vi "SRV_Sensor Streaming Sensors Off.vi"(0 "Previous Streaming Cfg-Cmds":T1[](array[typedef]) {"Calculated Sensors Array"."Parsed Formula"."Y Values" format="%.2f"; "Calculated Sensors Array"."Sensor Config"."Register" format="%.0x"; "Calculated Sensors Array"."Sensor Config"."I2C Address" format="%.0x"; "Calculated Sensors Array"."Sensor Config"."Sample Period (ms)" min=10 max=60000 step=1; "Calculated Sensors Array"."Sensor Config"."Digital Mask" format="%.0x"; "Calculated Sensors Array"."Sensor Config"."Channel" format="%.0x"; "Parsed Formula"."Y Values" format="%.2f"; "Sensor Config"."Register" format="%.0x"; "Sensor Config"."I2C Address" format="%.0x"; "Sensor Config"."Sample Period (ms)" min=10 max=60000 step=1; "Sensor Config"."Digital Mask" format="%.0x"; "Sensor Config"."Channel" format="%.0x"}, 11 "error in (no error)":errorcluster) -> (6 "Streaming Cfg-Cmds OFF":T1[](array[typedef]) {"Calculated Sensors Array"."Parsed Formula"."Y Values" format="%.2f"; "Calculated Sensors Array"."Sensor Config"."Register" format="%.0x"; "Calculated Sensors Array"."Sensor Config"."I2C Address" format="%.0x"; "Calculated Sensors Array"."Sensor Config"."Sample Period (ms)" min=10 max=60000 step=1; "Calculated Sensors Array"."Sensor Config"."Digital Mask" format="%.0x"; "Calculated Sensors Array"."Sensor Config"."Channel" format="%.0x"; "Parsed Formula"."Y Values" format="%.2f"; "Sensor Config"."Register" format="%.0x"; "Sensor Config"."I2C Address" format="%.0x"; "Sensor Config"."Sample Period (ms)" min=10 max=60000 step=1; "Sensor Config"."Digital Mask" format="%.0x"; "Sensor Config"."Channel" format="%.0x"}, 15 "error out":errorcluster)   [LabVIEW 2009]
uses:
  SRV_Sensor Config-Command Cluster.ctl
  SRV_Sensor Config Cluster.ctl
  SRV_Sensor Analog-Digital.ctl
  SRV_Sensor Sampling Mode.ctl
  SRV_Sensor View Config Cluster.ctl
  SRV_Sensors Names.ctl
  SRV_Sensor PicoC Shared Var Type.ctl
  SRV_Sensor Number of Bytes.ctl
  SRV_Sensor Integer Word Type.ctl
  SRV_Calculated Sensor Cfg.ctl
panel:
  # "operator"
  # "register1"
  # "register2"
  # "operator"
  # "register1"
  # "register2"
  # "operator"
  # "register1"
  # "register2"
  # "operator"
  # "register1"
  # "register2"
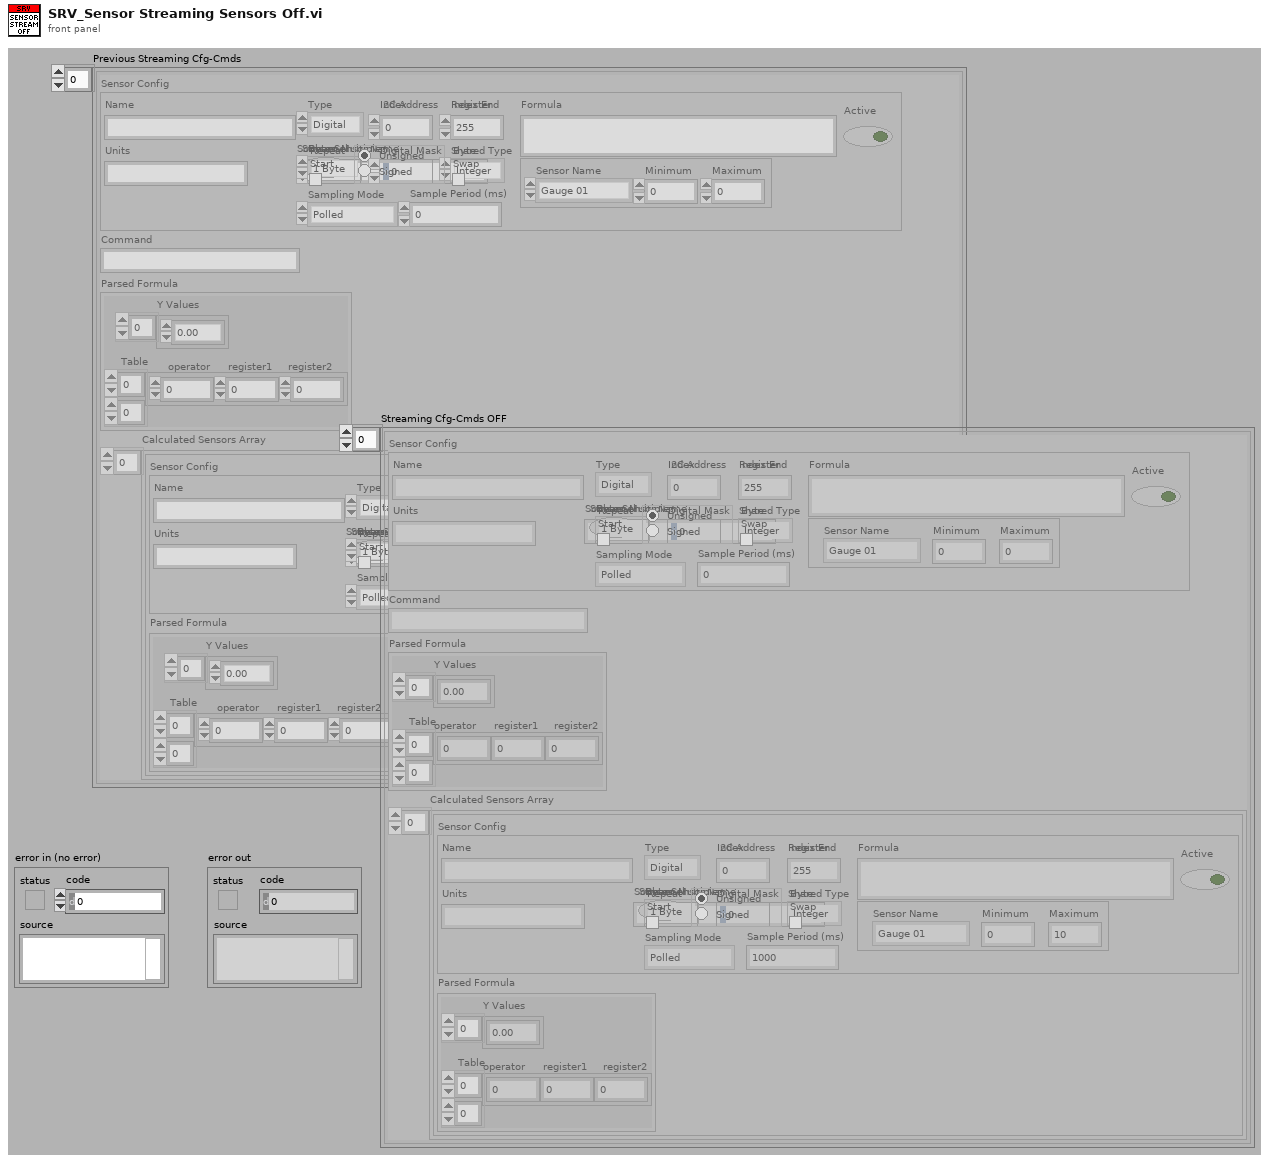
[diagram p1: front panel]
types:
  T1 = typedef "SRV_Sensor Config-Command Cluster.ctl" = cluster{"Sensor Config":T2, "Command":string, "Parsed Formula":cluster{"Table":i32[][], "Y Values":dbl[]}, "Calculated Sensors Array":T10[]}
  T2 = typedef "SRV_Sensor Config Cluster.ctl" = cluster{"Name":string, "A/D":T3, "I2C Address":u8, "Register":u8, "Channel":u8, "Digital Mask":u16, "Units":string, "Sampling Mode":T4, "Sample Period (ms)":u32, "Formula":string, "Sensor View Config":T5, "Active":bool, "PicoC Shared Var Type":T7, "Index":u8, "Stream Multiple?":bool, "Index End":u8, "Bytes":T8, "Source Sensor Name":string, "Repeat Start":bool, "Integer Word Type":T9, "Byte Swap":bool}
  T3 = typedef "SRV_Sensor Analog-Digital.ctl" = enum16{"Digital", "Analog", "PicoC Shared", "Calculated"}
  T4 = typedef "SRV_Sensor Sampling Mode.ctl" = enum16{"Polled", "Streaming"}
  T5 = typedef "SRV_Sensor View Config Cluster.ctl" = cluster{"Sensor Name":T6, "Minimum":dbl, "Maximum":dbl}
  T6 = typedef "SRV_Sensors Names.ctl" = enum16{"Gauge 01", "Gauge 02", "Gauge 03", "Gauge 04", "Meter 01", "Meter 02", "Meter 03", "Meter 04", "Numeric 01", "Numeric 02", "Numeric 03", "Numeric 04", "Numeric 05", "Numeric 06", "Numeric 07", "Numeric 08", "Boolean 01", "Boolean 02", "Boolean 03", "Boolean 04", "Boolean 05", "Boolean 06", "Boolean 07", "Boolean 08", "Boolean 09", "Boolean 10", "Boolean 11", "Boolean 12", "Boolean 13", "Boolean 14", "Boolean 15", "Boolean 16", "Boolean 17", "Boolean 18", "Boolean 19", "Boolean 20", "Boolean 21", "Boolean 22", "Boolean 23", "Boolean 24", "Boolean 25", "Boolean 26", "Boolean 27", "Boolean 28", "Boolean 29", "Boolean 30", "Boolean 31", "Boolean 32"}
  T7 = typedef "SRV_Sensor PicoC Shared Var Type.ctl" = enum16{"String", "Integer", "Float"}
  T8 = typedef "SRV_Sensor Number of Bytes.ctl" = enum16{"1 Byte", "2 Bytes"}
  T9 = typedef "SRV_Sensor Integer Word Type.ctl" = enum32{"Unsigned", "Signed"}
  T10 = typedef "SRV_Calculated Sensor Cfg.ctl" = cluster{"Sensor Config":T2, "Parsed Formula":cluster{"Table":i32[][], "Y Values":dbl[]}}
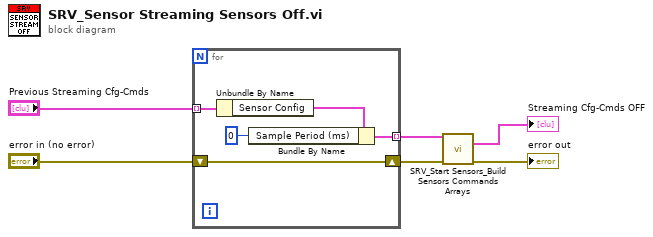
[diagram p0: block diagram]
diagram:
  n1 = for {
    tunnel: "Previous Streaming Cfg-Cmds" -> [w10] mode=indexing
    shift-right: [w8] -> w3
    shift-left: "error in (no error)" -> [w8]
    tunnel: [w7] -> w4 mode=indexing
    n2 = Unbundle By Name(w10) -> ("Sensor Config"=w9:T2)
    n3 = Bundle By Name(cluster=w9, "Sample Period (ms)"=u32 0 ("Sensor Config.Sample Period (ms)")) -> (w7:T2)
  }
  n4 = call "SRV_Start Sensors_Build Sensors Commands Arrays.vi"("Sensors Config"=w4, "error in (no error)"=w3) -> ("Active Streaming Cfg-Commands"=→"Streaming Cfg-Cmds OFF":T1[], "error out"=→"error out":errorcluster)  [unwired: 9 in, 3 out]
